vi "ramp.vi"(4 "channels (0)":string[](array[string])=["0,1,2"], 6 "device (1)":i32, 7 "points":i32, 8 "last value":dbl[](array[numeric]) format="%.2f", 9 "first value":dbl[](array[numeric]) format="%.2f", 10 "ramp time (s)":sgl format="%.2f") -> (3 "ramp array":sgl[][](array[numeric]) format="%.2f")   [LabVIEW 2010]
uses:
  AO Write (scaled array).vi
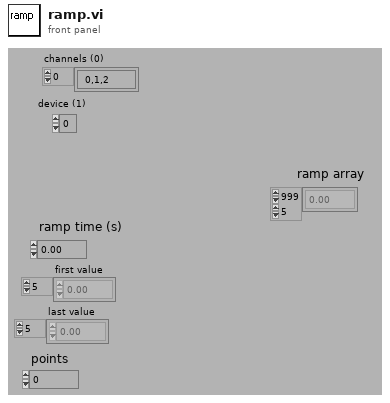
[diagram p1: front panel]
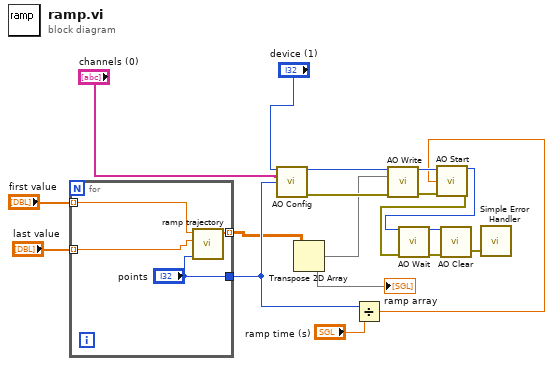
[diagram p0: block diagram]
diagram:
  n1 = for {
    tunnel: [w22] -> w2 mode=indexing
    tunnel: "last value" -> [w21] mode=indexing
    tunnel: ["points"] -> w4
    tunnel: "first value" -> [w19] mode=indexing
    n2 = call "ramp trajectory.vi"("points"="points", "end (volts)"=w21, "start (volts)"=w19) -> ("ramp"=w22:sgl[])  [unwired: 8 in]
  }
  n3 = call "AO Config.vi"("device (1)"="device (1)", "channels (0)"="channels (0)", "buffer size (1000 updates)"=w4) -> ("taskID"=w13:u32, "error out"=w8:errorcluster)  [unwired: 10 in, 1 out]
  n4 = Transpose 2D Array(2D array=w2) -> (transposed array=w1:sgl[][])
  "ramp array" <- w1
  n5 = Divide(x=w4, y="ramp time (s)") -> (x/y=w5:sgl)
  n6 = call-poly "AO Write.vi"("taskID in"=w13, "scaled data"=w1, "error in (no error)"=w8) -> ("taskID out"=w11:u32, "error out"=w12:errorcluster)  [unwired: 8 in, 3 out]
  n7 = call "AO Start.vi"("taskID in"=w11, "update rate (1000 updates/sec)"=w5, "error in (no error)"=w12) -> ("taskID out"=w18:u32, "error out"=w17:errorcluster)  [unwired: 10 in, 1 out]
  n8 = call "AO Wait.vi"("taskID in"=w18, "error in (no error)"=w17) -> ("taskID out"=w14:u32, "error out"=w15:errorcluster)  [unwired: 12 in]
  n9 = call "AO Clear.vi"("error in (no error)"=w15, "taskID in"=w14) -> ("error out"=w16:errorcluster)  [unwired: 4 in, 1 out]
  n10 = call <vilib>:"Simple Error Handler.vi"("error in (no error)"=w16) -> ()  [unwired: 4 in, 5 out]
